vi "FromMicroToBase.vi"(11 "u":dbl format="%#_13g") -> (3 "base":dbl)   [LabVIEW 2014]
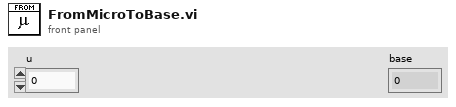
[diagram p1: front panel]
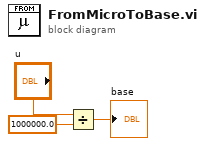
[diagram p0: block diagram]
diagram:
  n1 = Divide(x="u", y=1000000.0) -> (x/y=→"base":dbl)
